vi "Drag-on Subvi.vi"(0 "?":bool) -> ()   [LabVIEW 2013]
panel:
  # "DRAG ON?"
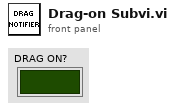
[diagram p1: front panel]
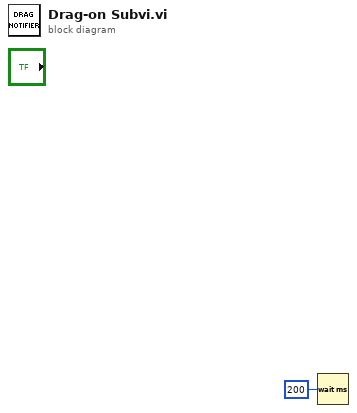
[diagram p0: block diagram]
diagram:
  n1 = Wait (ms)(milliseconds to wait=u32 200) -> ()  [unwired: 1 out]
